vi "FPGA_laser_control_Qudi_.vi"() -> ()   [LabVIEW 2015]
uses:
  <vilib>/Platform/TimedLoop/XDataNode/timing_clust.ctl
  <vilib>/Platform/TimedLoop/XDataNode/nitl_modes.ctl
  <vilib>/Platform/TimedLoop/XDataNode/wakeup.ctl
  <vilib>/rvi/FXPMathLib/basic elements/FxpIntAccumulator/subVIs/nifxpmath_IntAccumulator_SimConfig.ctl
  <vilib>/rvi/eio/common/nirviEmuTemplateMethod_errors.vi
  <vilib>/rvi/Emulation/niFpgaGetClockAttributes.vi
  <vilib>/rvi/Emulation/niFpgaSctlEmulationGetInTimedLoop.vi
  <vilib>/rvi/Emulation/niFpgaEmulationReportErrorSimple.vi
  <vilib>/rvi/Analysis/common/codeGenErrors/XNode/niFpgaXNodeCodeGenErrorHandle.vi
  <vilib>/rvi/Emulation/niFpgaCriticalErrorInLSC.vi
  <vilib>/rvi/FXPMathLib/basic elements/FxpIntAccumulator/simVIs/DllFxpIntAccumulator_sub.vi
  <vilib>/eio/EIONode/EIONode.xnode
  <vilib>/rvi/Analysis/measure/dc-rms/XNode/niFpgaDC-RMS.xnode
  <vilib>/Platform/TimedLoop/XDataNode/XDataNode.xnode
  <vilib>/rvi/FXPMathLib/basic elements/FxpIntAccumulator/XNode/nifxpmath_IntAccumulator.xnode
  <vilib>/Platform/TimedLoop/XDataNode/XDNodeRunTimeDep.lvlib
panel:
  in  "Task":bool
  out "I":i16
  out "Y":i16
  out "X":i16
  out "Duration_ms":u32
  in  "Integration_time_us":u32=100 caption="Count(uSec)"
  in  "488":i16
  in  "405":i16
  in  "640":i16
  in  "561":i16
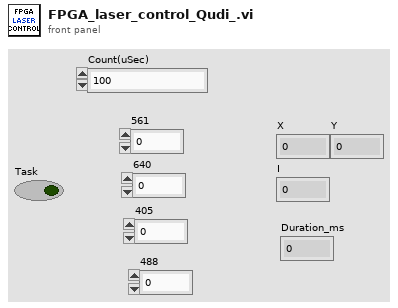
[diagram p1: front panel]
types:
  T1 = typedef "XDNodeRunTimeDep.lvlib/timing_clust.ctl" = cluster{"Expected End [f-1]":u64, "Actual End [f-1]":u64, "Finished Late? [f-1]":bool, "Expected End [i-1]":u64, "Actual End [i-1]":u64, "Finished Late? [i-1]":bool, "Expected Start [i]":u64, "Actual Start [i]":u64, "Expected Start [f]":u64, "Actual Start [f]":u64, "Source Name":string, "Structure Name":string, "Period":i64, "Deadline":i64, "Offset":i64, "Start":i64, "Priority":i32, "Timeout":i32, "Mode":T2, "Wakeup Reason":T3, "Error":errorcluster, "Source Type":string, "Secondary Source Type":string, "Global End Time":u64, "Global Start Time":u64, "Frame Duration":u64, "Iteration Duration":u64, "Assigned CPU":i32, "I/O Scan Engine Mode":u32}
  T2 = typedef "XDNodeRunTimeDep.lvlib/nitl_modes.ctl" = enum32{"No Change", "Process missed periods, maintain original phase", "Discard missed periods, maintain original phase", "Process missed periods, ignore original phase", "Discard missed periods, ignore original phase"}
  T3 = typedef "XDNodeRunTimeDep.lvlib/wakeup.ctl" = enum32{"Normal", "Aborted", "Asynchronous wakeup", "Timing source error", "Timed loop error", "Timeout"}
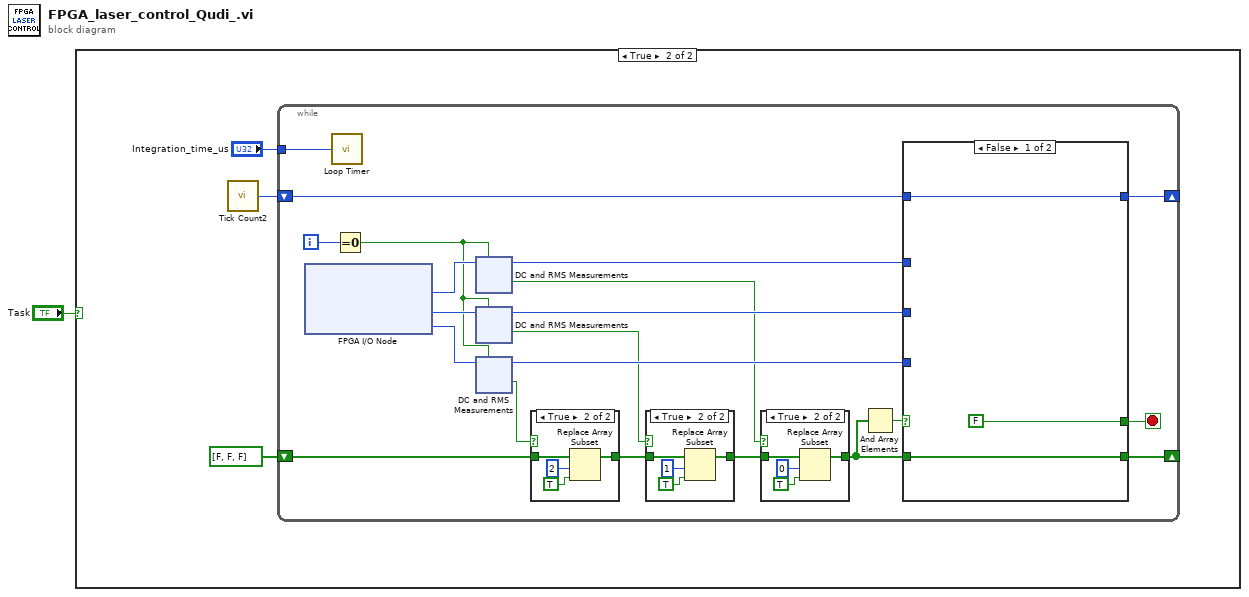
[diagram p0: block diagram]
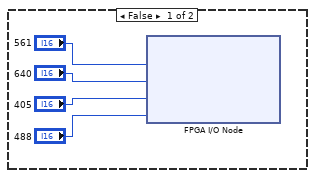
[diagram p2: hidden frame]
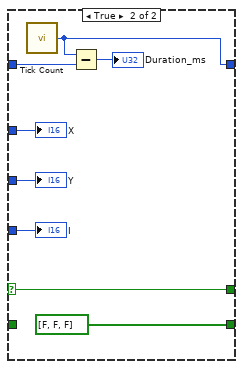
[diagram p6: hidden frame]
diagram:
  n1 = case shown="True" "Task" {
    frame False {
      n2 = xnode "FPGA I/O Node"("Connector0/AO0"="561", "Connector0/AO1"="640", "Connector0/AO2"="405", "Connector0/AO3"="488") -> ()  [unwired: 4 in, 4 out]
    }
    frame True {
      n3 = call "Tick Count2"() -> ("Tick Count(mSec)"=w6:u32)
      n4 = while {
        shift-right: [w13] -> _
        shift-left: bool[] [FALSE, FALSE, FALSE] ("initialized array") -> [w21]
        shift-right: [w11] -> _
        shift-left: w6 -> [w12]
        tunnel: "Integration_time_us" -> [w10]
        i -> [w28]
        stop <- w9 stop-if-true
        n5 = xnode "FPGA I/O Node"() -> ("Connector0/AI0"=w29:i16, "Connector0/AI1"=w26:i16, "Connector0/AI2"=w25:i16)  [unwired: 3 in, 3 out]
        n6 = call "Loop Timer"("Count(uSec)"=w10) -> ()  [unwired: 1 out]
        n7 = Equal To 0?(x=w28) -> (x = 0?=w22:bool)
        n8 = xnode "DC and RMS Measurements"("input data"=w29, "reset"=w22) -> ("DC"=w27:i16, "output valid"=w16:bool)
        n9 = xnode "DC and RMS Measurements"("input data"=w26, "reset"=w22) -> ("DC"=w24:i16, "output valid"=w17:bool)
        n10 = xnode "DC and RMS Measurements"("input data"=w25, "reset"=w22) -> ("DC"=w23:i16, "output valid"=w18:bool)
        n11 = case shown="True" w18 {
          tunnel: w21 -> [w35 w38]
          tunnel: [w35 w36] -> w20
          frame False {
          }
          frame True {
            n12 = Replace Array Subset(array=w38, new element=TRUE, index=2) -> (w36:bool[])
          }
        }
        n13 = case shown="True" w17 {
          tunnel: w20 -> [w40 w43]
          tunnel: [w40 w41] -> w19
          frame False {
          }
          frame True {
            n14 = Replace Array Subset(array=w43, new element=TRUE, index=1) -> (w41:bool[])
          }
        }
        n15 = case shown="True" w16 {
          tunnel: [w30 w32] -> w14
          tunnel: w19 -> [w30 w31]
          frame False {
          }
          frame True {
            n16 = Replace Array Subset(array=w31, new element=TRUE, index=0) -> (w32:bool[])
          }
        }
        n17 = And Array Elements(Boolean array=w14) -> (logical AND=w15:bool)
        n18 = case shown="False" w15 {
          selector: w15 -> [_ w51]
          tunnel: w27 -> [_ w50]
          tunnel: w24 -> [_ w48]
          tunnel: w23 -> [_ w49]
          tunnel: w14 -> [w47 _]
          tunnel: [w47 bool[] [FALSE, FALSE, FALSE] ("initialized array")] -> w13
          tunnel: w12 -> [w46 w54]
          tunnel: [w46 w52] -> w11
          tunnel: [FALSE w51] -> w9
          frame False {
          }
          frame True {
            n19 = call "Tick Count"() -> ("Tick Count(mSec)"=w52:u32)
            n20 = Subtract(x=w52, y=w54) -> (x-y=→"Duration_ms":u32)
            "X" <- w50
            "Y" <- w48
            "I" <- w49
          }
        }
      }
    }
  }
